vi "Service Wrapper.vi"(8 "error in (no error)":errorcluster, 11 "Pub Sub Message Channel in":refnum<class "Pub Sub Message Channel.lvclass">) -> (0 "error out":errorcluster, 3 "Pub Sub Message Channel out":refnum<class "Pub Sub Message Channel.lvclass">)   [LabVIEW 2020, in "Actor Pub Sub Channels.lvlib" / "Pub Sub Message Channel.lvclass"]
uses:
  Pub Sub Message Channel.lvclass
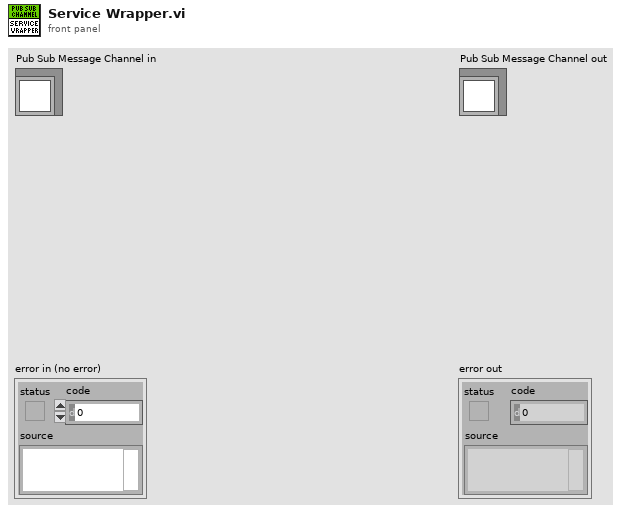
[diagram p1: front panel]
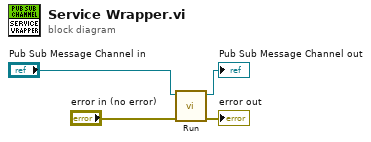
[diagram p0: block diagram]
diagram:
  n1 = call-dynamic "Run.vi"("error in (no error)"="error in (no error)", "Pub Sub Message Channel in"="Pub Sub Message Channel in") -> ("error out"=→"error out":errorcluster, "Pub Sub Message Channel out"=→"Pub Sub Message Channel out":refnum<class "Pub Sub Message Channel.lvclass">)  [unwired: 8 in]
